vi "Save Recall Instrument Settings.vi"(8 "error in (no error)":errorcluster, 9 "Memory Location (0)":dbl min=0.0 max=100.0 format="%#_0f", 10 "Save Recall Settings (0:Save)":u16(ring) items=["Save", "Recall"], 11 "VISA resource name":refnum<visa-resource-name>) -> (0 "error out":errorcluster, 3 "VISA resource name out":refnum<visa-resource-name>)   [LabVIEW 2018, in "BK Precision 8600 Series.lvlib"]
doc: "Saves or recalls instrument settings to or from a specified memory location."
uses:
  <instrlib>/BK Precision 8600 Series/BK Precision 8600 Series.lvlib
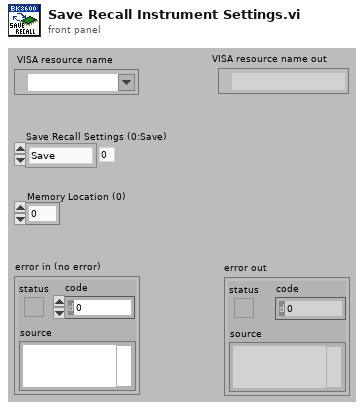
[diagram p1: front panel]
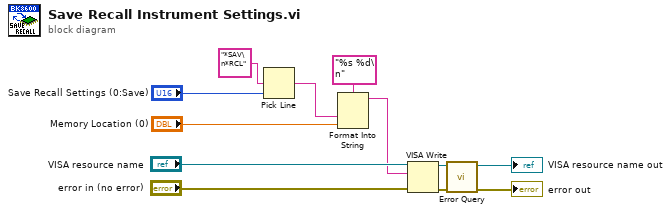
[diagram p0: block diagram]
diagram:
  n1 = Pick Line(multi-line string="*SAV\n*RCL", line index="Save Recall Settings (0:Save)") -> (output string=w9:string)  [unwired: 1 in]
  n2 = Format Into String(format string="%s %d\n", w9, "Memory Location (0)") -> (resulting string=w1:string)  [unwired: 2 in, 1 out]
  n3 = VISA Write(VISA resource name="VISA resource name", write buffer=w1, error in (no error)="error in (no error)") -> (VISA resource name out=w6:refnum<visa-resource-name>, error out=w5:errorcluster)  [unwired: 1 out]
  n4 = call <instrlib>:"Error Query.vi"("error in (no error)"=w5, "VISA resource name"=w6) -> ("error out"=→"error out":errorcluster, "VISA resource name out"=→"VISA resource name out":refnum<visa-resource-name>)  [unwired: 6 in, 2 out]
